vi "Extended Register Write Long.vi"(0 "instrument handle in":refnum<k15>, 1 "Bus Number":i32, 5 "Slave Address":T3=12 format="%02x", 7 "Register Address":T2 format="%02x", 9 "Register Data":T1[](array[typedef]) format="%02x", 11 "error in (no error)":errorcluster) -> (4 "instrument handle out":refnum<k15>, 15 "error out":errorcluster)   [LabVIEW 2018, in "MIPI RFFE API.lvlib"]
uses:
  MIPI RFFE API.lvlib
  Slave Address.ctl
  Register Address.ctl
  Register Data.ctl
  RegWriteExtLong/RFFE RegWriteExtLong Command.lvclass
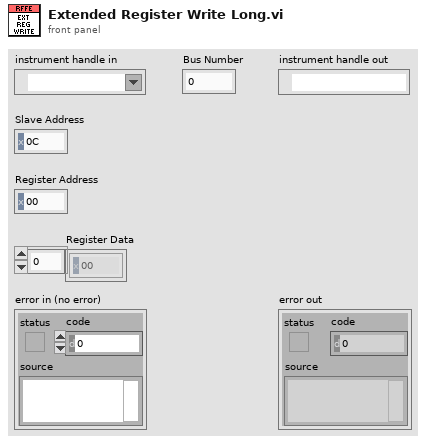
[diagram p1: front panel]
types:
  T1 = typedef "MIPI RFFE API.lvlib/Register Data.ctl" = u8
  T2 = typedef "MIPI RFFE API.lvlib/Register Address.ctl" = u16
  T3 = typedef "MIPI RFFE API.lvlib/Slave Address.ctl" = u8
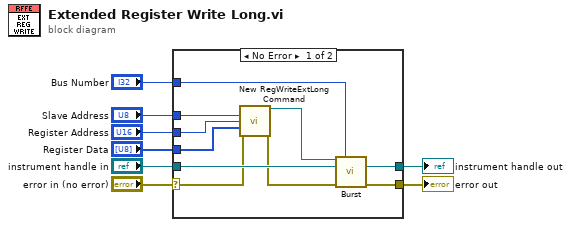
[diagram p0: block diagram]
diagram:
  n1 = case shown="No Error" "error in (no error)" {
    selector: "error in (no error)" -> [w15 w19]
    tunnel: "instrument handle in" -> [w18 w20]
    tunnel: [w17 w20] -> w7
    tunnel: "Slave Address" -> [w10 _]
    tunnel: "Register Address" -> [w9 _]
    tunnel: "Register Data" -> [w12 _]
    tunnel: [w13 w19] -> w2
    tunnel: "Bus Number" -> [w11 _]
    frame No Error {
      n2 = call "New RegWriteExtLong Command.vi"("Slave Address"=w10, "Register Address"=w9, "Register Data"=w12, "error in (no error)"=w15) -> ("RFFE RegWriteExt Command out"=w16:refnum<class "RFFE RegWriteExtLong Command.lvclass">, "error out"=w14:errorcluster)  [unwired: 10 in]
      n3 = call-dynamic "Burst.vi"("RFFE Command in"=w16, "Bus Number"=w11, "instrument handle in"=w18, "error in (no error)"=w14) -> ("instrument handle out"=w17:refnum<k15>, "error out"=w13:errorcluster)  [unwired: 9 in, 1 out]
    }
    frame Error {
    }
  }
  "instrument handle out" <- w7
  "error out" <- w2
